vi "ingest.tabular_begin.vi"(8 "error in (no error)":errorcluster, 11 "Client in":refnum<class "Client.lvclass">) -> (0 "error out":errorcluster, 2 "TabularIngestStaging":refnum<class "TabularIngestStaging.lvclass">, 3 "Client out":refnum<class "Client.lvclass">)   [LabVIEW 2020, in "Client.lvclass"]
uses:
  Client.lvclass
  Client.lvclass/Client.ctl
  client.lvlib
  TabularIngestStaging/TabularIngestStaging.lvclass
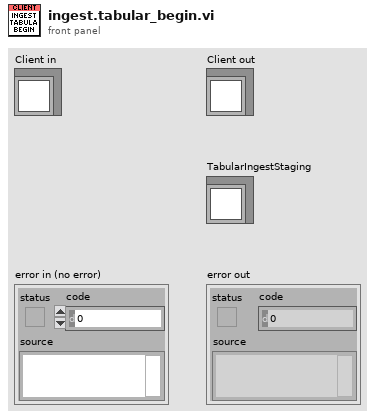
[diagram p1: front panel]
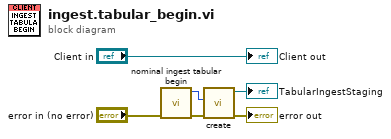
[diagram p0: block diagram]
diagram:
  n1 = call "nominal ingest tabular begin.vi"("error in (no error)"="error in (no error)") -> ("error out"=w3:errorcluster, "out_staging out"=w4:i32)  [unwired: 8 in, 1 out]
  n2 = call "create.vi"("error in (no error)"=w3, "handle"=w4) -> ("error out"=→"error out":errorcluster, "TabularIngestStaging"=→"TabularIngestStaging":refnum<class "TabularIngestStaging.lvclass">)  [unwired: 8 in]
  "Client out" <- "Client in"
